vi "HOST Leaderboard.vi"() -> ()   [LabVIEW 2026]
uses:
  Leaderboard Announcement.ctl
panel:
  in  "Cancel Button":bool
  out "1 Player Leaderboard":string[][](table)
  out "2 Player Leaderboard":string[][](table)
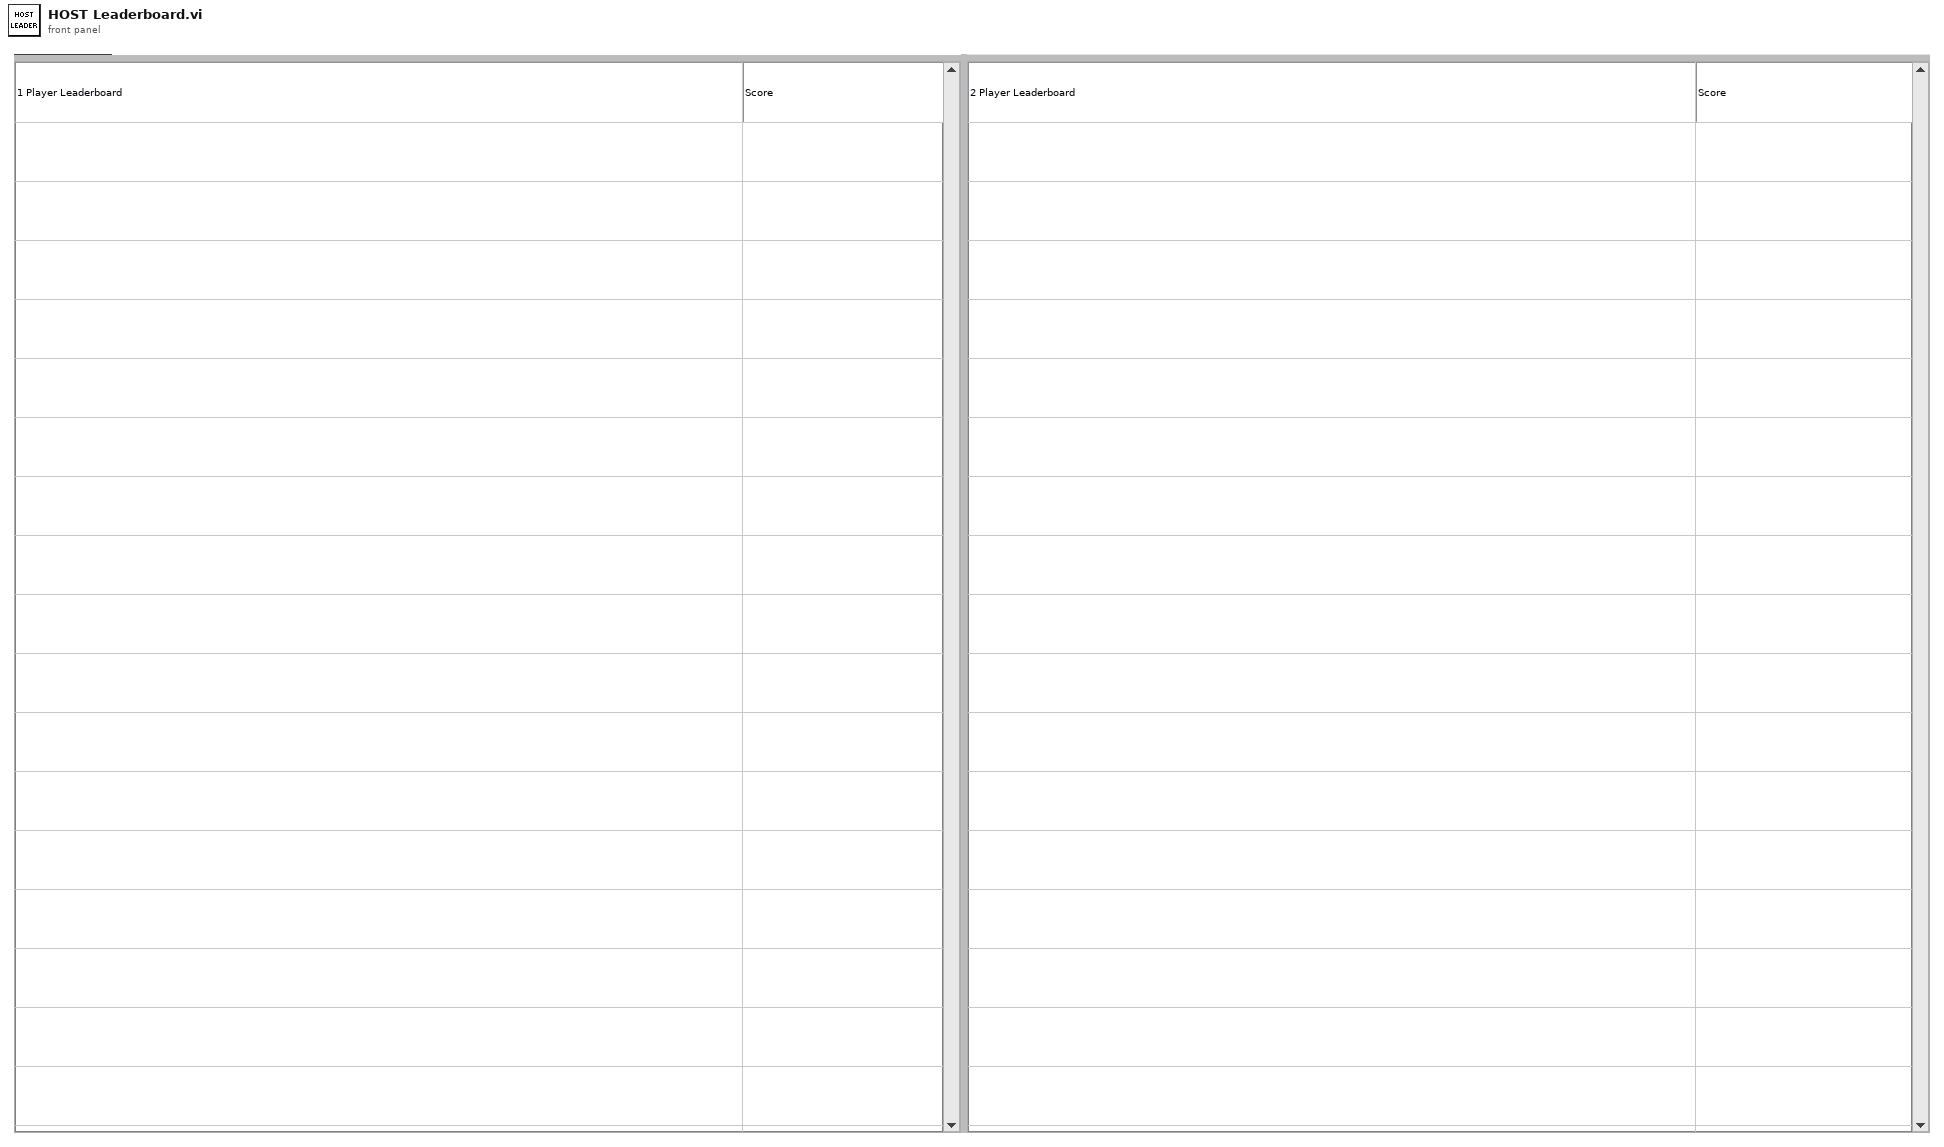
[diagram p1: front panel]
types:
  T1 = cluster{"Score P1":u16, "Player 1 Name":string}[]
  T2 = typedef "Leaderboard Announcement.ctl" = cluster{"Player 1 Name":string, "Score P1":u16, "Player 1 Name 2":string, "Score P1 2":u16}
  T3 = cluster{"Score P1 2":u16, "Player 1 Name 2":string}
  T4 = cluster{"Score P1 2":u16, "Player 1 Name 2":string}[]
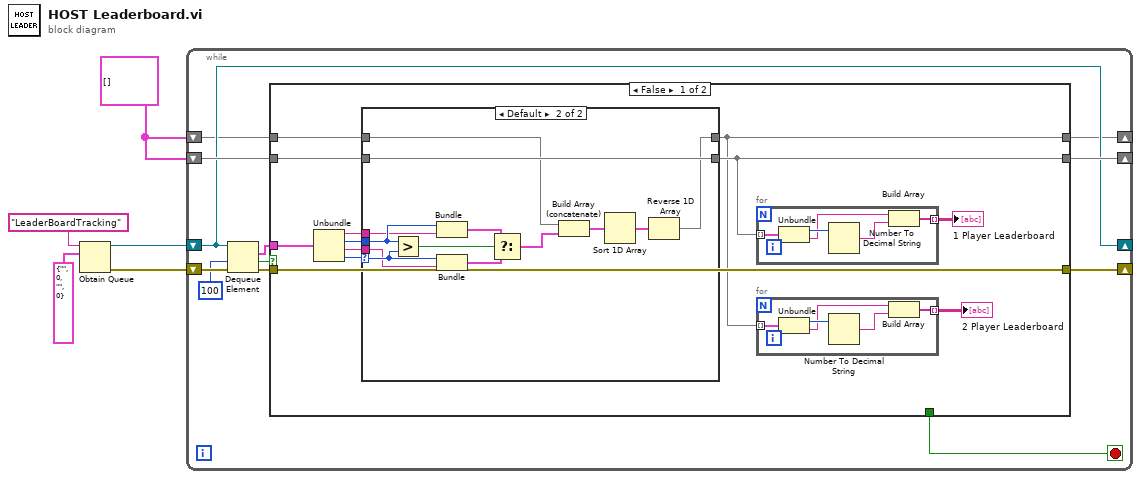
[diagram p0: block diagram]
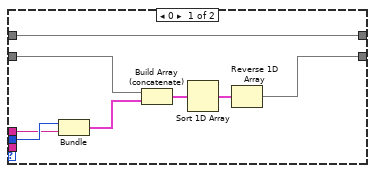
[diagram p2: hidden frame]
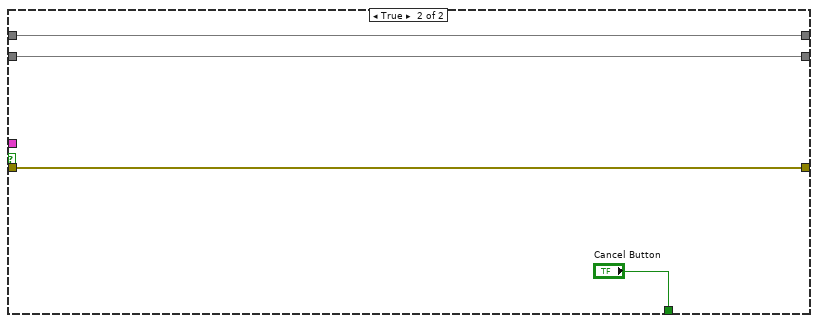
[diagram p3: hidden frame]
diagram:
  w1 = T1 []
  n1 = Obtain Queue(name (unnamed)="LeaderBoardTracking", element data type=T2 {"Player 1 Name"="", "Score P1"=0, "Player 1 Name 2"="", "Score P1 2"=0} ("output cluster")) -> (queue out=w3:refnum<queue>, error out=w2:errorcluster)  [unwired: 3 in, 1 out]
  n2 = while {
    shift-right: [w8] -> _
    shift-left: w3 -> [w8]
    shift-right: [w10] -> _
    shift-left: w2 -> [w17]
    shift-right: [w14] -> _
    shift-left: w1 -> [w13]
    shift-right: [w7] -> _
    shift-left: w1 -> [w6]
    stop <- w11 stop-if-true
    n3 = Dequeue Element(queue=w8, timeout in ms (-1)=100, error in (no error)=w17) -> (element=w16:T2, timed out?=w15:bool, error out=w9:errorcluster)  [unwired: 1 out]
    n4 = case shown="False" w15 {
      tunnel: w16 -> [w29 _]
      tunnel: [w23 w64] -> w14
      tunnel: w13 -> [w24 w64]
      tunnel: [_ "Cancel Button"] -> w11
      tunnel: [w21 w63] -> w10
      tunnel: w9 -> [w21 w63]
      tunnel: [w18 w61] -> w7
      tunnel: w6 -> [w19 w61]
      frame False {
        n5 = Unbundle(w29) -> ("Player 1 Name"=w26:string, "Score P1"=w27:u16, "Player 1 Name 2"=w25:string, "Score P1 2"=w28:u16)
        n6 = case shown="Default" w28 {
          selector: w28 -> [_ w54]
          tunnel: w27 -> [w47 w56]
          tunnel: w26 -> [w46 w55]
          tunnel: w25 -> [_ w53]
          tunnel: [w41 w60] -> w23
          tunnel: w24 -> [w43 w60]
          tunnel: [w40 w57] -> w18
          tunnel: w19 -> [w40 w48]
          frame 0 {
            n7 = Bundle("Score P1"=w47, "Player 1 Name"=w46) -> (w45:cluster{"Score P1":u16, "Player 1 Name":string})  [unwired: 1 in]
            n8 = Build Array (concatenate)(w43, w45) -> (w44:T1)
            n9 = Sort 1D Array(array=w44) -> (sorted array=w42:T1)
            n10 = Reverse 1D Array(array=w42) -> (reversed array=w41:T1)
          }
          frame Default {
            n11 = Greater?(x=w56, y=w54) -> (0:w50:bool)
            n12 = Bundle("Score P1"=w56, "Player 1 Name"=w55) -> (w52:cluster{"Score P1":u16, "Player 1 Name":string})  [unwired: 1 in]
            n13 = Bundle("Score P1 2"=w54, "Player 1 Name 2"=w53) -> (w51:T3)  [unwired: 1 in]
            n14 = Select(t=w52, s=w50, f=w51) -> (s? t:f=w49:T3)
            n15 = Build Array (concatenate)(w48, w49) -> (w59:T4)
            n16 = Sort 1D Array(array=w59) -> (sorted array=w58:T4)
            n17 = Reverse 1D Array(array=w58) -> (reversed array=w57:T4)
          }
        }
        n18 = for {
          tunnel: w23 -> [w39] mode=indexing
          tunnel: [w35] -> w22 mode=indexing
          n19 = Unbundle(w39) -> ("Score P1"=w38:u16, "Player 1 Name"=w37:string)
          n20 = Number To Decimal String(number=w38) -> (decimal integer string=w36:string)  [unwired: 1 in]
          n21 = Build Array(w37, w36) -> (w35:string[])
        }
        "1 Player Leaderboard" <- w22
        n22 = for {
          tunnel: w18 -> [w34] mode=indexing
          tunnel: [w30] -> w20 mode=indexing
          n23 = Unbundle(w34) -> ("Score P1 2"=w33:u16, "Player 1 Name 2"=w32:string)
          n24 = Number To Decimal String(number=w33) -> (decimal integer string=w31:string)  [unwired: 1 in]
          n25 = Build Array(w32, w31) -> (w30:string[])
        }
        "2 Player Leaderboard" <- w20
      }
      frame True {
      }
    }
  }
